vi "ritter flow.vi"(8 "error in (no error)":errorcluster, 11 "VISA in":refnum<visa-resource-name>) -> (0 "error out":errorcluster, 1 "flow (ltr/hr)":dbl, 2 "flow (cuft/hr)":dbl, 3 "VISA out":refnum<visa-resource-name>)   [LabVIEW 2023]
doc: "This vi returns the current flow through the Ritter gasmeter."
panel:
  out "reading":string
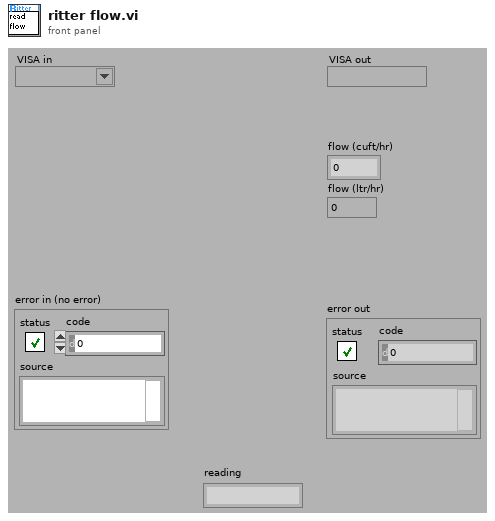
[diagram p1: front panel]
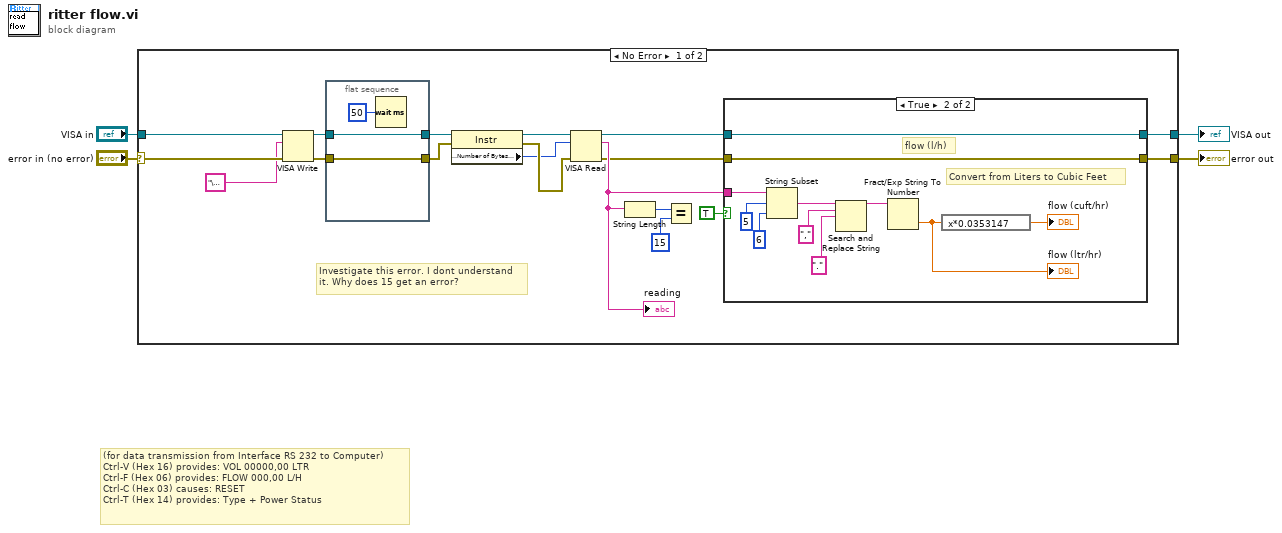
[diagram p0: block diagram]
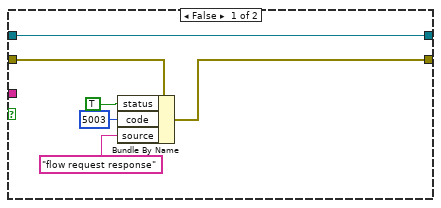
[diagram p2: hidden frame]
diagram:
  # "(for data transmission from Interface RS 232 to Computer)\nCtrl-V (Hex 16) provides: VOL 00000,00 LTR\nCtrl-F (Hex 06) provides: FLOW 000,00 L/H\nCtrl-C (Hex 03) causes: RESET\nCtrl-T (Hex 14) provides: Type + Power Status"
  n1 = case shown="No Error" "error in (no error)" {
    selector: "error in (no error)" -> [w14 w43]
    tunnel: [w9 w43] -> w4
    tunnel: "VISA in" -> [w15 w44]
    tunnel: [w7 w44] -> w2
    frame No Error {
      # "Investigate this error. I dont understand\nit. Why does 15 get an error?"
      n2 = VISA Write(VISA resource name=w15, write buffer="\u0006", error in (no error)=w14) -> (VISA resource name out=w21:refnum<visa-resource-name>, error out=w22:errorcluster)  [unwired: 1 out]
      n3 = flat-sequence {
        tunnel: w22 -> [w42]
        tunnel: [w42] -> w20
        tunnel: w21 -> [w41]
        tunnel: [w41] -> w19
        frame #0 {
          n4 = Wait (ms)(milliseconds to wait=u32 50) -> ()  [unwired: 1 out]
        }
      }
      n5 = property class="Instr"(reference=w19, error in=w20) -> (reference out=w18:refnum<visa-resource-name>, error out=w17:errorcluster, "Serial Settings:Number of Bytes at Serial Port"=w16:u32)
      n6 = VISA Read(VISA resource name=w18, byte count=w16, error in (no error)=w17) -> (VISA resource name out=w8:refnum<visa-resource-name>, read buffer=w13:string, error out=w10:errorcluster)  [unwired: 1 out]
      "reading" <- w13
      n7 = String Length(string=w13) -> (length=w12:i32)
      n8 = Equal?(x=w12, y=15) -> ()  [unwired: 1 out]
      n9 = case shown="True" TRUE {
        tunnel: w13 -> [_ w33]
        tunnel: w10 -> [w27 w32]
        tunnel: [w23 w32] -> w9
        tunnel: w8 -> [w28 w31]
        tunnel: [w28 w31] -> w7
        frame False {
          n10 = Bundle By Name(cluster=w27, "status"=TRUE, "code"=5003, "source"="flow request response") -> (w23:errorcluster)
        }
        frame True {
          # "Convert from Liters to Cubic Feet"
          # "flow (l/h)"
          n11 = String Subset(string=w33, offset (0)=5, length (rest)=6 ("length (rest)")) -> (substring=w35:string)
          n12 = Search and Replace String(input string=w35, search string=",", replace string="." ("replace string (\"\")")) -> (result string=w34:string)  [unwired: 5 in, 3 out]
          n13 = Fract/Exp String To Number(string=w34) -> (number=w30:dbl)  [unwired: 3 in, 1 out]
          "flow (ltr/hr)" <- w30
          n14 = expression code="x*0.0353147"(w30) -> (→"flow (cuft/hr)":dbl)
        }
      }
    }
    frame Error {
    }
  }
  "error out" <- w4
  "VISA out" <- w2
